vi "Copy_Argument_For_ID.vi"(1 "Value":string, 2 "Argument":string, 3 "API ID":string, 4 "Input Sequence":cluster{string, string[], dbl[], dbl}[](array[cluster])) -> (0 "Output Sequence":cluster{string, string[], dbl[], dbl}[](array[cluster]))   [LabVIEW 2011]
doc: "This VI will copy a given argument and its text value to all commands in the sequence with the given ID."
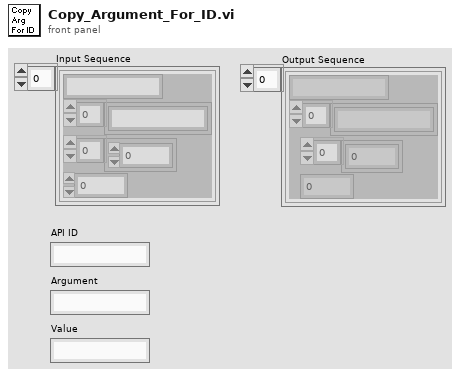
[diagram p1: front panel]
types:
  T1 = cluster{string, "Argument List Out":string[], dbl[], dbl}
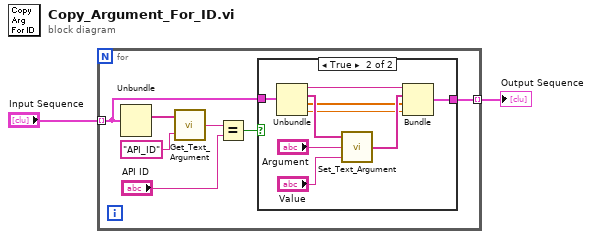
[diagram p0: block diagram]
diagram:
  n1 = for {
    tunnel: "Input Sequence" -> [w4] mode=indexing
    tunnel: [w3] -> w1 mode=indexing
    n2 = Unbundle(w4) -> (w9:string[])  [unwired: 3 out]
    n3 = call "Get_Text_Argument.vi"("Argument"="API_ID", "Argument List"=w9) -> ("Text"=w7:string)
    n4 = Equal?(x=w7, y="API ID") -> (x = y?=w5:bool)
    n5 = case shown="True" w5 {
      tunnel: w4 -> [w10 w19]
      tunnel: [w10 w11] -> w3
      frame False {
      }
      frame True {
        n6 = Unbundle(w19) -> (w12:string, w18:string[], w14:dbl[], w13:dbl)
        n7 = call "Set_Text_Argument.vi"("Text"="Value", "Argument"="Argument", "Argument List In"=w18) -> ("Argument List Out"=w15:string[])
        n8 = Bundle(w12, "Argument List Out"=w15, w14, w13) -> (w11:T1)  [unwired: 1 in]
      }
    }
  }
  "Output Sequence" <- w1
